vi "Convert to Interface State.vi"(8 "error in (no error)":errorcluster, 11 "Instrument State in":T2) -> (0 "error out":errorcluster, 3 "Instrument State out":variant)   [LabVIEW 2020, in "Omega Platinum Series Plugin.lvlib" / "Remote Connection Manager.lvlib"]
doc: "Converts the internal instrument state into the instrument state representation used by the remote system."
uses:
  Remote Connection Manager.lvlib
  Instrument Manager/Instrument State.ctl
  Typedefs/Remote Temperature Controller State.ctl
  Omega Platinum Series Plugin.lvlib
  Instrument Manager/Instrument Manager.lvlib
panel:
  out "Remote Temperature Controller State":T1
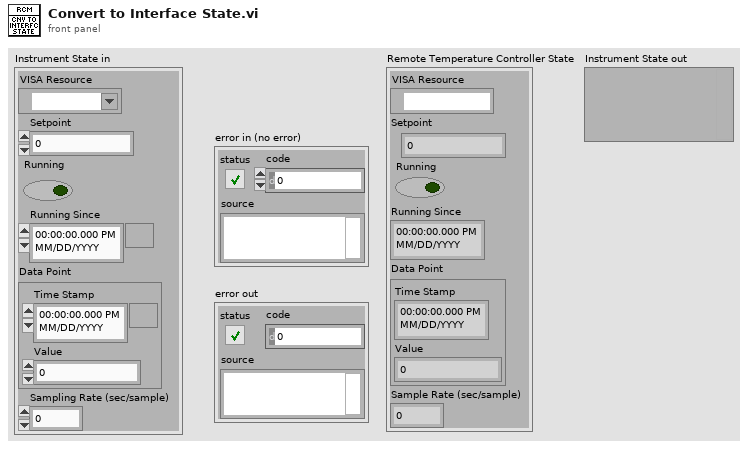
[diagram p1: front panel]
types:
  T1 = typedef "Omega Platinum Series Plugin.lvlib/Remote Temperature Controller State.ctl" = cluster{"VISA Resource":refnum<visa-resource-name>, "Setpoint":dbl, "Running":bool, "Running Since":timestamp, "Data Point":cluster{"Time Stamp":timestamp, "Value":dbl}, "Sample Rate (sec/sample)":dbl}
  T2 = typedef "Omega Platinum Series Plugin.lvlib/Instrument Manager.lvlib/Instrument State.ctl" = cluster{"VISA Resource":refnum<visa-resource-name>, "Setpoint":dbl, "Running":bool, "Running Since":timestamp, "Data Point":cluster{"Time Stamp":timestamp, "Value":dbl}, "Sampling Rate (sec/sample)":dbl}
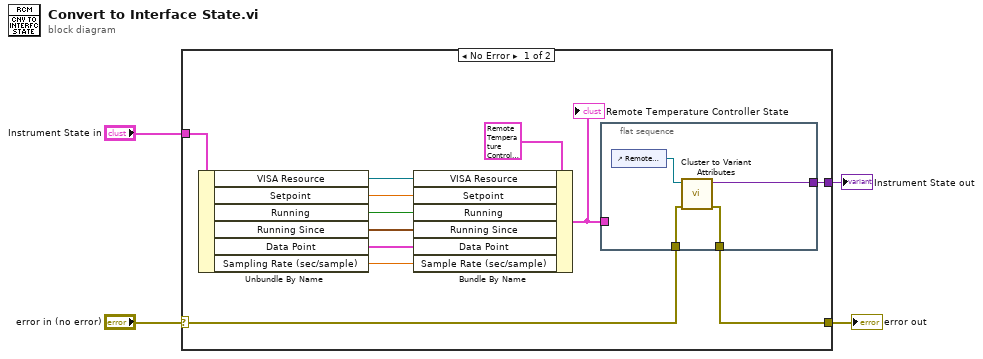
[diagram p0: block diagram]
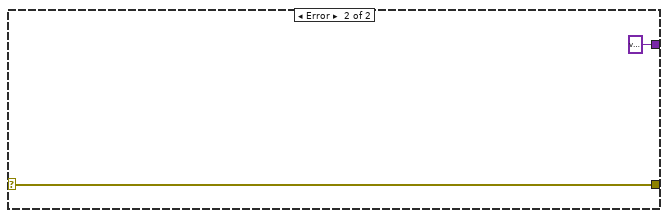
[diagram p2: hidden frame]
diagram:
  n1 = case shown="No Error" "error in (no error)" {
    selector: "error in (no error)" -> [w8 w22]
    tunnel: "Instrument State in" -> [w15 _]
    tunnel: [w7 w22] -> w2
    tunnel: [w6 variant ("Variant out")] -> w1
    frame No Error {
      n2 = Unbundle By Name(w15) -> ("VISA Resource"=w14:refnum<visa-resource-name>, "Setpoint"=w13:dbl, "Running"=w12:bool, "Running Since"=w11:timestamp, "Data Point"=w10:cluster{"Time Stamp":timestamp, "Value":dbl}, "Sampling Rate (sec/sample)"=w9:dbl)
      n3 = Bundle By Name(cluster=T1 {"VISA Resource"="", "Setpoint"=0.0, "Running"=FALSE, "Running Since"=timestamp(0 s since 1904-01-01), "Data Point"={"Time Stamp"=timestamp(0 s since 1904-01-01), "Value"=0.0}, "Sample Rate (sec/sample)"=0.0} ("Instrument State"), "VISA Resource"=w14, "Setpoint"=w13, "Running"=w12, "Running Since"=w11, "Data Point"=w10, "Sample Rate (sec/sample)"=w9) -> (w5:T1)
      "Remote Temperature Controller State" <- w5
      n4 = flat-sequence {
        tunnel: w8 -> [w19]
        tunnel: [w18] -> w7
        tunnel: [w17] -> w6
        tunnel: w5 -> [_]
        frame #0 {
          n5 = control-ref of="Remote Temperature Controller State"() -> (w20:refnum<vi>)
          n6 = call "Cluster to Variant Attributes.vi"("error in (no error)"=w19, "Cluster in"=w20) -> ("error out"=w18:errorcluster, "Variant out"=w17:variant)  [unwired: 8 in]
        }
      }
    }
    frame Error {
    }
  }
  "error out" <- w2
  "Instrument State out" <- w1
